vi "Reset.vi"(11 "Test Suite In":refnum<class "LUnit Test Suite.lvclass">) -> (3 "Test Suite Out":refnum<class "LUnit Test Suite.lvclass">)   [LabVIEW 2020, in "LUnit Test Suite.lvclass"]
doc: "Resets results and current test case."
uses:
  LUnit Test Suite.lvclass
  LUnit Test Suite.lvclass/LUnit Test Suite.ctl
  Result Types/Suite Results/Test Suite Result.ctl
  Result Types/Assertion Result/Public/TypeDefs/Status.ctl
  Result Types/Case Result/Test Case Result.ctl
  Result Types/Method Result/Method Result.ctl
  Rewrite Project/Result/Status.ctl
  Result Types/Assertion Result/Assertion Result.ctl
  Result Types/Assertion Result/Public/TypeDefs/Assertion Type.ctl
  Result Types/Assertion Result/Assertion Result.lvlib
  Result Types/Case Result/Test Case Result.lvlib
  Result Types/Suite Results/Test Suite Result.lvlib
  Rewrite Project/Result/Result.lvlib
  Result Types/Method Result/Method Result.lvlib
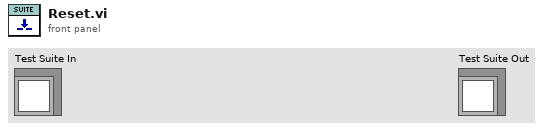
[diagram p1: front panel]
types:
  T1 = typedef "Test Suite Result.lvlib/Test Suite Result.ctl" = cluster{"Test Suite ID":string, "Name":string, "Hostname":string, "Status":T2, "Execution time":dbl, "Start Time":timestamp, "Case Results":T3[]}
  T2 = typedef "Assertion Result.lvlib/Status.ctl" = enum16{"Pass", "Fail", "Error", "Skipped", "Setup Error", "Broken", "Teardown Error"}
  T3 = typedef "Test Case Result.lvlib/Test Case Result.ctl" = map{string, T4}
  T4 = typedef "Method Result.lvlib/Method Result.ctl" = cluster{"Test Case":string, "Test Method Name":string, "Status":T5, "Assertion Results":T6[], "Execution time":dbl, "Result String":string}
  T5 = typedef "Result.lvlib/Status.ctl" = enum16{"Pass", "Fail", "Error", "Skipped", "Setup Error", "Broken", "Teardown Error"}
  T6 = typedef "Assertion Result.lvlib/Assertion Result.ctl" = cluster{"Status":T5, "Message":string, "Description":string, "Assertion Type":T7}
  T7 = typedef "Result.lvlib/Assertion Type.ctl" = enum16{"None", "Pass", "Fail", "Skip", "Pass if Equal", "Fail if Equal", "Pass if Error", "Fail if Error", "Pass if", "Fail if"}
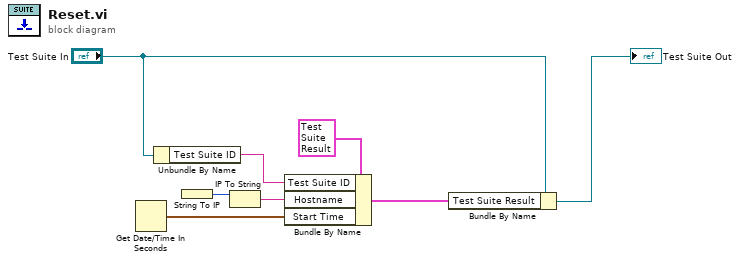
[diagram p0: block diagram]
diagram:
  n1 = Get Date/Time In Seconds() -> (seconds since 1Jan1904=w2:timestamp)
  n2 = Unbundle By Name("Test Suite In") -> ("Test Suite ID"=w6:string)
  n3 = String To IP() -> (0:w5:u32)  [unwired: 1 in]
  n4 = IP To String(2:w5) -> (0:w3:string)  [unwired: 1 in]
  n5 = Bundle By Name(cluster=T1 {"Test Suite ID"="", "Name"="", "Hostname"="", "Status"=enum."Pass", "Execution time"=0.0, "Start Time"=timestamp(0 s since 1904-01-01), "Case Results"=[]} ("Test Suite Result"), "Test Suite ID"=w6, "Hostname"=w3, "Start Time"=w2) -> (w1:T1)
  n6 = Bundle By Name(cluster="Test Suite In", "Test Suite Result"=w1) -> (→"Test Suite Out":refnum<class "LUnit Test Suite.lvclass">)
